vi "Simulator SNA Resample Complex Waveform (Single Shot Linear Interpolation).vi"(7 "open interval? (T)":bool=TRUE, 8 "error in (no error)":errorcluster, 9 "t0":timestamp=timestamp(-9223372036854775808 s since 1904-01-01) format="%<%.4X>T", 10 "dt":dbl=1.0 format="%.2p", 11 "waveform in":waveform(cdb)) -> (0 "error out":errorcluster, 1 "used t0":timestamp=timestamp(-9223372036854775808 s since 1904-01-01) format="%<%.4X>T", 3 "resampled waveform out":waveform(cdb), 4 "t0 adjusted warning":bool)   [LabVIEW 2011]
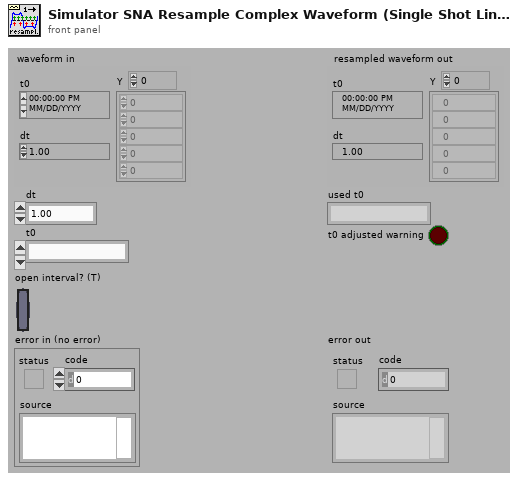
[diagram p1: front panel]
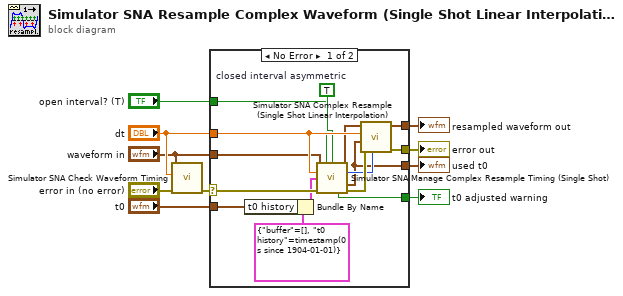
[diagram p0: block diagram]
diagram:
  n1 = call "Simulator SNA Check Waveform Timing.vi"("error in (no error)"="error in (no error)", "dt"="dt", "signal in"="waveform in") -> ("error out"=w8:errorcluster)  [unwired: 8 out]
  n2 = case shown="No Error" w8 {
    selector: w8 -> [w24 w26]
    tunnel: [w25 w26] -> w10
    tunnel: "dt" -> [w23 _]
    tunnel: "waveform in" -> [w22 _]
    tunnel: "open interval? (T)" -> [w15 _]
    tunnel: "t0" -> [w11 _]
    tunnel: [w14 _] -> w3
    tunnel: [w13 _] -> w2
    tunnel: [w12 _] -> w1
    frame No Error {
      w18 = TRUE  # closed interval asymmetric
      n3 = Bundle By Name(cluster=cluster{"buffer":cdb[], "t0 history":timestamp} {"buffer"=[], "t0 history"=timestamp(0 s since 1904-01-01)} ("state info in"), "t0 history"=w11) -> (w16:cluster{"buffer":cdb[], "t0 history":timestamp})
      n4 = call "Simulator SNA Manage Complex Resample Timing (Single Shot).vi"("waveform in"=w22, "open interval? (T)"=w15, "closed interval asymmetric"=w18, "dt"=w23, "state info in"=w16, "error in"=w24) -> ("waveform to be processed"=w19:waveform(cdb), "#elements"=w20:i32, "used t0"=w13:timestamp, "t0 adjusted warning"=w12:bool, "error out"=w21:errorcluster)  [unwired: 5 out]
      n5 = call "Simulator SNA Complex Resample (Single Shot Linear Interpolation).vi"("#elements"=w20, "error in"=w21, "t0"=w13, "dt"=w23, "waveform in"=w19) -> ("error out"=w25:errorcluster, "resampled waveform out"=w14:waveform(cdb))  [unwired: 5 out]
    }
    frame Error {
    }
  }
  "error out" <- w10
  "t0 adjusted warning" <- w1
  "used t0" <- w2
  "resampled waveform out" <- w3
